vi "Display.vi"(11 "Error_In":errorcluster) -> (4 "Waveform Chart":dbl(graph), 15 "Error_Out":errorcluster)   [LabVIEW 2023]
doc: "This is the main Chart module to show the record output."
uses:
  Controls/Operation.ctl
  Controls/Event_Data.ctl
  Controls/Event_Data_and_Parameter.ctl
  LV2/UE_C_LV2.vi
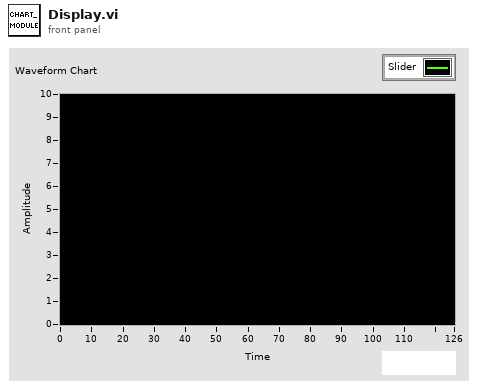
[diagram p1: front panel]
types:
  T1 = typedef "Event_Data_and_Parameter.ctl" = cluster{"Event_Data":dbl[], "Generate_Event":bool, "Playback?":bool, "Index":i32}
  T2 = typedef "Event_Data.ctl" = cluster{"Event_Data":dbl, "PlayBack?":bool}
  T3 = typedef "Operation.ctl" = enum16{"Create_UE", "Generate_UE", "Destroy_UE", "Get_UE_Reference"}
  T4 = enum32{"Bad", "Idle", "Run top level", "Running"}
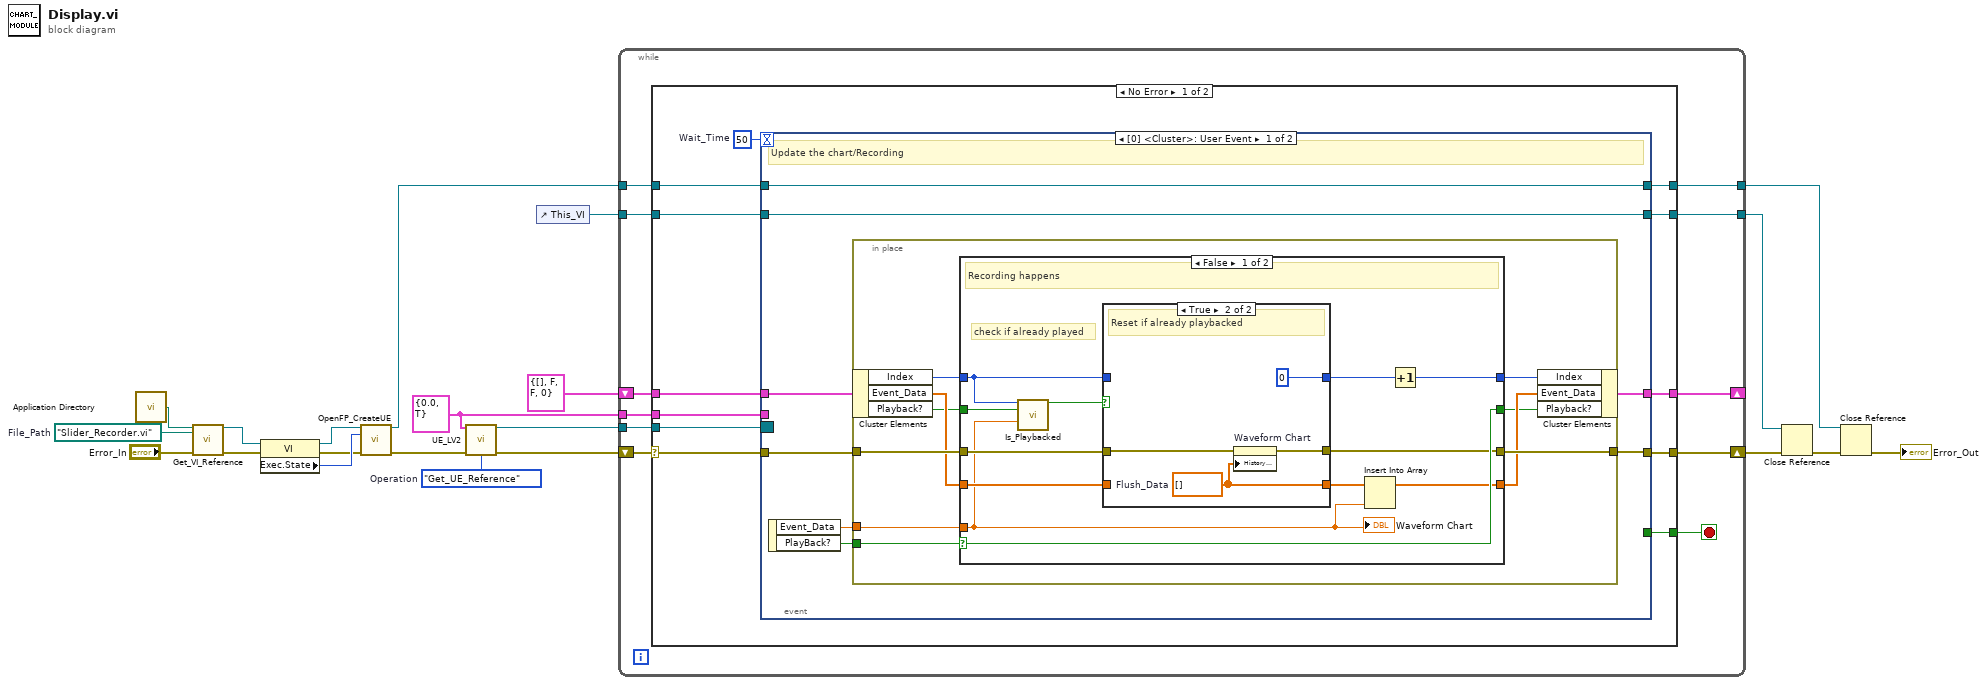
[diagram p0: block diagram]
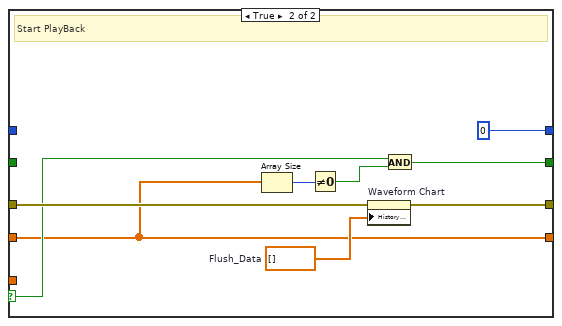
[diagram p3: hidden frame]
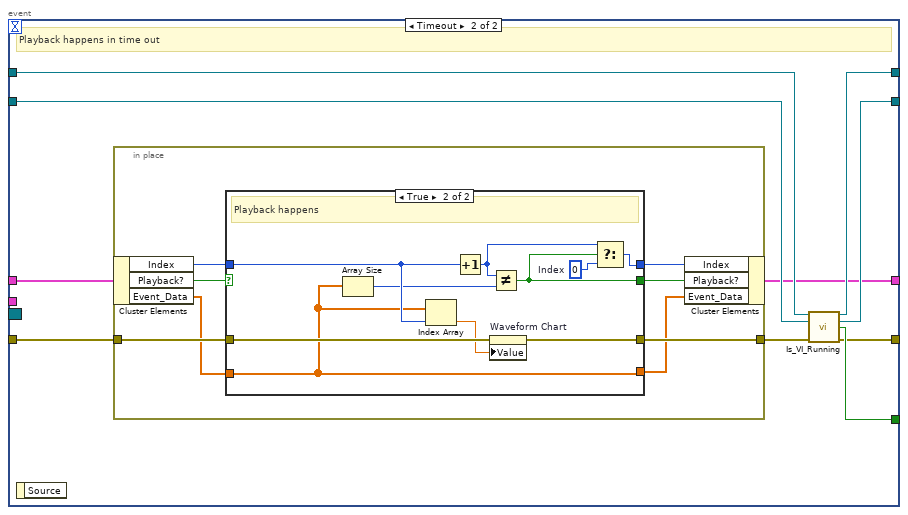
[diagram p4: hidden frame]
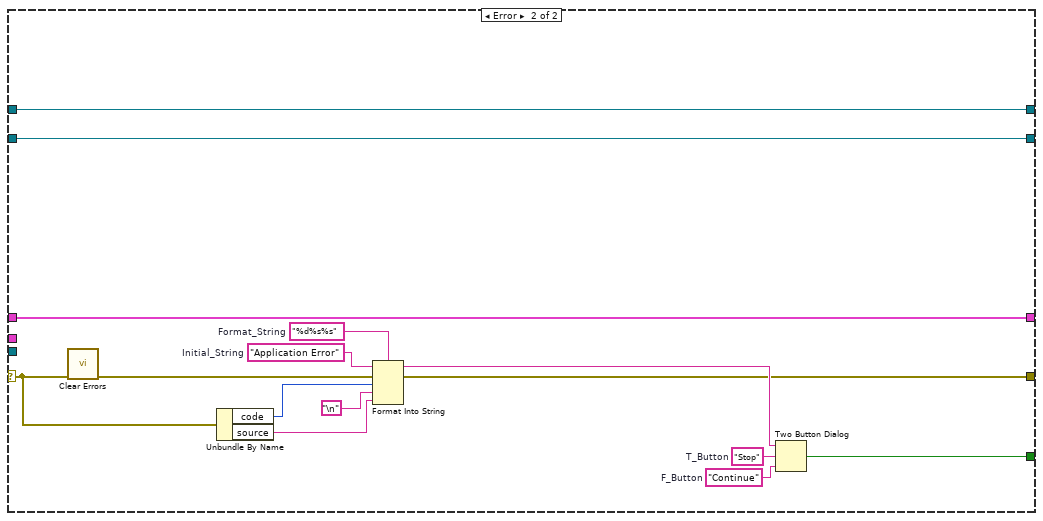
[diagram p6: hidden frame]
diagram:
  w1 = T2 {"Event_Data"=0.0, "PlayBack?"=TRUE} ("Event_Data")
  w13 = Operation."Get_UE_Reference"  # Operation
  w16 = path "Slider_Recorder.vi"  # File_Path
  n1 = call <vilib>:"Application Directory.vi"() -> ("Application Directory"=w17:path)
  n2 = call "Get_VI_Reference.vi"("Application_Directory"=w17, "File_Path"=w16, "Error_In"="Error_In") -> ("VI_Reference"=w15:refnum<vi>, "Error_Out"=w18:errorcluster)  [unwired: 11 in]
  n3 = property class="VI"(reference=w15, error in=w18) -> (reference out=w14:refnum<vi>, error out=w20:errorcluster, "Exec.State"=w21:T4)
  n4 = call "OpenFP_CreateUE.vi"("VI_Reference_In"=w14, "Exec.State"=w21, "Error_In"=w20) -> ("VI_Reference_Out"=w9:refnum<vi>, "Error_Out"=w12:errorcluster)  [unwired: 11 in]
  n5 = call-poly "UE_LV2.vi"("Event_Data"=w1, "Error_In"=w12, "Operation"=w13) -> ("Event_Reference"=w10:refnum<event-registration>, "Error_Out"=w11:errorcluster)  [unwired: 11 in]
  n6 = control-ref of="This_VI"() -> (w8:refnum<vi>)
  n7 = while {
    shift-right: [w28] -> _
    shift-left: T1 {"Event_Data"=[], "Generate_Event"=FALSE, "Playback?"=FALSE, "Index"=0} ("Event_Data_and_Parameter") -> [w29]
    tunnel: w10 -> [w27]
    tunnel: w9 -> [w26]
    tunnel: w8 -> [w25]
    tunnel: [w24] -> w4
    tunnel: [w23] -> w3
    tunnel: w1 -> [w22]
    shift-right: [w31] -> w7
    shift-left: w11 -> [w32]
    stop <- w30 stop-if-true
    n8 = case shown="No Error" w32 {
      selector: w32 -> [w43 w124]
      tunnel: [w42 w127] -> w31
      tunnel: [w41 w123] -> w30
      tunnel: w29 -> [w40 w137]
      tunnel: [w34 w137] -> w28
      tunnel: w27 -> [w39 _]
      tunnel: w26 -> [w38 w136]
      tunnel: w25 -> [w37 w135]
      tunnel: [w36 w135] -> w24
      tunnel: [w35 w136] -> w23
      tunnel: w22 -> [w33 _]
      frame No Error {
        w44 = 50  # Wait_Time
        n9 = event shown="[0] <Cluster>: User Event" {
          selector: w39 -> [_ _]
          dyn-events: _ -> [_ _]
          timeout: w44 -> [_ _]
          tunnel: w43 -> [w51 w100]
          tunnel: [w52 w94] -> w42
          tunnel: [_ w98] -> w41
          tunnel: w40 -> [w46 w92]
          tunnel: w38 -> [w50 w97]
          tunnel: w37 -> [w49 w95]
          tunnel: [w49 w93] -> w36
          tunnel: [w50 w96] -> w35
          tunnel: [w45 w91] -> w34
          tunnel: w33 -> [_ _]
          event User Event {
            # "Update the chart/Recording"
            n10 = event-data() -> ("Event_Data"=w48:dbl, "PlayBack?"=w47:bool)  [unwired: 1 in]
            n11 = in-place {
              in-place-border: [w62] -> w52
              in-place-border: w51 -> [w61]
              in-place-border: w48 -> [w58]
              in-place-border: w47 -> [w60]
              n12 = in-place-cluster #1(w46) -> ("Index"=w59:i32, "Event_Data"=w56:dbl[], "Playback?"=w55:bool)
              n13 = case shown="False" w60 {
                selector: w60 -> [w74 w87]
                tunnel: w56 -> [w72 w84]
                tunnel: [w69 w84] -> w54
                tunnel: w58 -> [w64 _]
                tunnel: [w68 w89] -> w62
                tunnel: w61 -> [w73 w90]
                tunnel: [w74 w85] -> w53
                tunnel: w59 -> [w66 _]
                tunnel: [w67 0] -> w57
                tunnel: w55 -> [w63 _]
                frame False {
                  # "check if already played"
                  # "Recording happens"
                  n14 = call "Is_Playbacked.vi"("Index"=w66, "Playback?"=w63, "Event_Data"=w64) -> ("Is_Playback"=w65:bool)  [unwired: 12 in]
                  n15 = case shown="True" w65 {
                    tunnel: w73 -> [w76 w80]
                    tunnel: [w76 w79] -> w68
                    tunnel: [w77 w78] -> w70
                    tunnel: w72 -> [w77 _]
                    tunnel: [w75 0] -> w71
                    tunnel: w66 -> [w75 _]
                    frame False {
                      # "Recording"
                    }
                    frame True {
                      w78 = dbl[] []  # Flush_Data
                      # "Reset if already playbacked"
                      n16 = property on="Waveform Chart" class="WFChart (strict)"(error in=w80, "History Data"=w78) -> (error out=w79:errorcluster)  [unwired: 1 in, 1 out]
                    }
                  }
                  n17 = Insert Into Array(array=w70, new element=w64) -> (w69:dbl[])  [unwired: 1 in]
                  n18 = Increment(x=w71) -> (x+1=w67:i32)
                  "Waveform Chart" <- w64
                }
                frame True {
                  w88 = dbl[] []  # Flush_Data
                  # "Start PlayBack"
                  n19 = Array Size(array=w84) -> (size(s)=w83:i32)
                  n20 = Not Equal To 0?(x=w83) -> (x != 0?=w82:bool)
                  n21 = property on="Waveform Chart" class="WFChart (strict)"(error in=w90, "History Data"=w88) -> (error out=w89:errorcluster)  [unwired: 1 in, 1 out]
                  n22 = And(x=w87, y=w82) -> (x .and. y?=w85:bool)
                }
              }
              n23 = in-place-cluster #1("Index"=w57, "Event_Data"=w54, "Playback?"=w53) -> (w45:T1)
            }
          }
          event Timeout {
            # "Playback happens in time out"
            n24 = event-data() -> ()  [unwired: 1 in, 1 out]
            n25 = in-place {
              in-place-border: w100 -> [w108]
              in-place-border: [w107] -> w99
              n26 = in-place-cluster #2(w92) -> ("Index"=w105:i32, "Playback?"=w106:bool, "Event_Data"=w104:dbl[])
              n27 = case shown="True" w106 {
                selector: w106 -> [w110 _]
                tunnel: w108 -> [w112 w121]
                tunnel: [w112 w122] -> w107
                tunnel: w104 -> [w111 w116]
                tunnel: [w111 w116] -> w102
                tunnel: [w110 w114] -> w101
                tunnel: [w109 w115] -> w103
                tunnel: w105 -> [w109 w119]
                frame False {
                }
                frame True {
                  w113 = 0  # Index
                  # "Playback happens"
                  n28 = Array Size(array=w116) -> (size(s)=w117:i32)
                  n29 = Index Array(array=w116, index=w119) -> (element=w120:dbl)
                  n30 = Increment(x=w119) -> (x+1=w118:i32)
                  n31 = property on="Waveform Chart" class="WFChart (strict)"(error in=w121, "Value"=w120) -> (error out=w122:errorcluster)  [unwired: 1 in, 1 out]
                  n32 = Not Equal?(x=w118, y=w117) -> (x != y?=w114:bool)
                  n33 = Select(t=w118, s=w114, f=w113) -> (s? t:f=w115:i32)
                }
              }
              n34 = in-place-cluster #2("Index"=w103, "Playback?"=w101, "Event_Data"=w102) -> (w91:T1)
            }
            n35 = call "Is_VI_Running.vi"("Other_VI_Reference_In"=w97, "This_VI_Reference_In"=w95, "Error_In"=w99) -> ("Other_VI_Reference_Out"=w96:refnum<vi>, "This_VI_Reference_Out"=w93:refnum<vi>, "Stop"=w98:bool, "Error_Out"=w94:errorcluster)  [unwired: 9 in]
          }
        }
      }
      frame Error {
        w130 = "%d%s%s"  # Format_String
        w131 = "Application Error"  # Initial_String
        w132 = "Stop"  # T_Button
        w133 = "Continue"  # F_Button
        n36 = call <vilib>:"Clear Errors.vi"("error in (no error)"=w124) -> ("error out"=w128:errorcluster)  [unwired: 5 in, 1 out]
        n37 = Unbundle By Name(w124) -> ("code"=w126:i32, "source"=w125:string)
        n38 = Format Into String(format string=w130, initial string=w131, error in=w128, w126, "\n" ("Line Feed Constant"), w125) -> (resulting string=w134:string, error out=w127:errorcluster)
        n39 = Two Button Dialog(message=w134, 1:w133, 2:w132) -> (T button?=w123:bool)
      }
    }
  }
  n40 = Close Reference(reference=w4, error in (no error)=w7) -> (error out=w5:errorcluster)
  n41 = Close Reference(reference=w3, error in (no error)=w5) -> (error out=→"Error_Out":errorcluster)
